vi "CU_writeQualityMeasure.vi"(8 "error in (no error)":errorcluster, 10 "ClassifierQualityMeasure in":T1, 11 "ClassifierClass in":refnum<class "ClassifierClass.lvclass">) -> (0 "error out":errorcluster, 3 "ClassifierClass out":refnum<class "ClassifierClass.lvclass">)   [LabVIEW 2016, in "Classifier.lvlib" / "ClassifierClass.lvclass"]
uses:
  ClassifierClass.lvclass
  CU_ClassifierQualityMeasure.ctl
  ClassifierClass.lvclass/ClassifierClass.ctl
  Classifier.lvlib
panel:
  # "This VI is a part of BCI Design library, http://www.ru-bci.org \nCopyright © 2020, Sotnikov Peter, All rights reserved. License: GNU GPLv3"
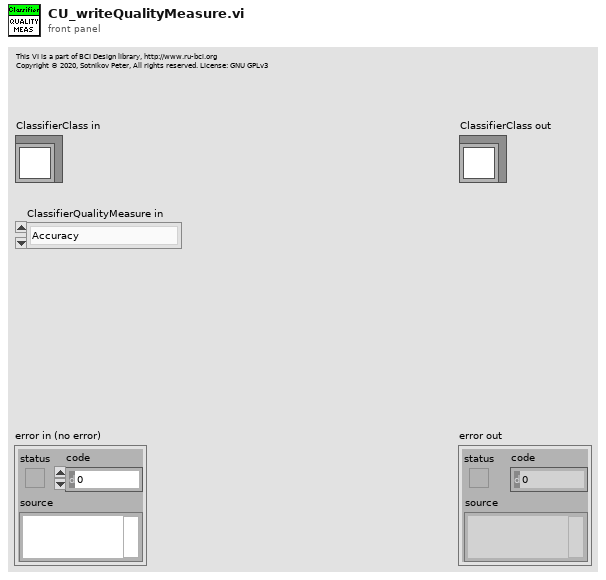
[diagram p1: front panel]
types:
  T1 = typedef "Classifier.lvlib/CU_ClassifierQualityMeasure.ctl" = enum16{"Accuracy", "Cohen's kappa"}
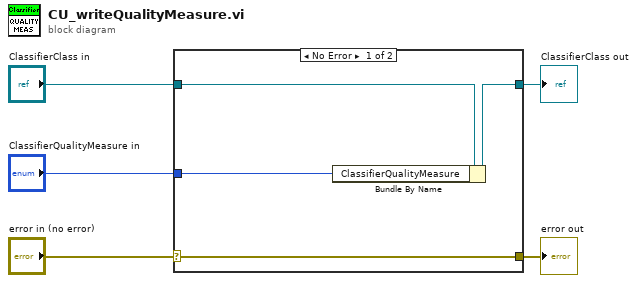
[diagram p0: block diagram]
diagram:
  n1 = case shown="No Error" "error in (no error)" {
    selector: "error in (no error)" -> [w9 w10]
    tunnel: [w9 w10] -> w4
    tunnel: [w7 w11] -> w2
    tunnel: "ClassifierClass in" -> [w8 w11]
    tunnel: "ClassifierQualityMeasure in" -> [w6 _]
    frame No Error {
      n2 = Bundle By Name(cluster=w8, "ClassifierQualityMeasure"=w6) -> (w7:refnum<class "ClassifierClass.lvclass">)
    }
    frame Error {
    }
  }
  "error out" <- w4
  "ClassifierClass out" <- w2
